vi "WFRepetitionsAssemble.vi"(9 "Repeat":i32=1 min=1, 10 "Interval (s)":dbl min=0.0, 11 "Delay (s)":dbl min=0.0) -> (3 "Repetitions":T1={"Delay (s)"=0.0, "Interval (s)"=0.0, "Repeat"=1} {"Interval (s)" min=0.0; "Delay (s)" min=0.0})   [LabVIEW 2013]
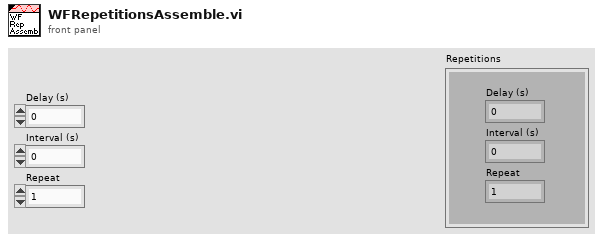
[diagram p1: front panel]
types:
  T1 = cluster{"Delay (s)":dbl, "Interval (s)":dbl, "Repeat":i32}
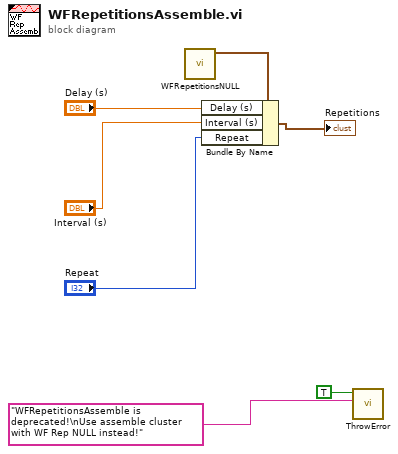
[diagram p0: block diagram]
diagram:
  n1 = call "WFRepetitionsNULL.vi"() -> ("Repetitions"=w7:T1)  [unwired: 11 in]
  n2 = Bundle By Name(cluster=w7, "Delay (s)"="Delay (s)", "Interval (s)"="Interval (s)", "Repeat"="Repeat") -> (→"Repetitions":T1)
  n3 = call "ThrowError.vi"("Error Message"="WFRepetitionsAssemble is deprecated!\nUse assemble cluster with WF Rep NULL instead!", "Error Input"=TRUE) -> ()  [unwired: 8 in, 2 out]
